vi "Register.vi"(5 "Color":T1={"Red"=0.0, "Green"=0.0, "Blue"=1.0, "Alpha"=1.0}, 6 "Point Size":sgl=10.0, 7 "Name":string, 8 "error in (no error)":errorcluster, 9 "Capacity":i32, 10 "Root Sence":refnum<vi>, 11 "Trace Drawer in":refnum<class "Trajectory Drawer.lvclass">) -> (0 "error out":errorcluster, 2 "Root Sence Out":refnum<vi>, 3 "Trace Drawer out":refnum<class "Trajectory Drawer.lvclass">)   [LabVIEW 2014, in "Trajectory Drawer.lvclass"]
uses:
  Trajectory Drawer.lvclass
  <vilib>/Utility/miscctls.llb/LVRGBAColorTypeDef.ctl
  Trajectory Drawer.lvclass/Trajectory Drawer.ctl
  <vilib>/picture/3D Picture Control/Object/Create Object (drawable with reference).vi
  <vilib>/picture/3D Picture Control/NI_3D Picture Control.lvlib
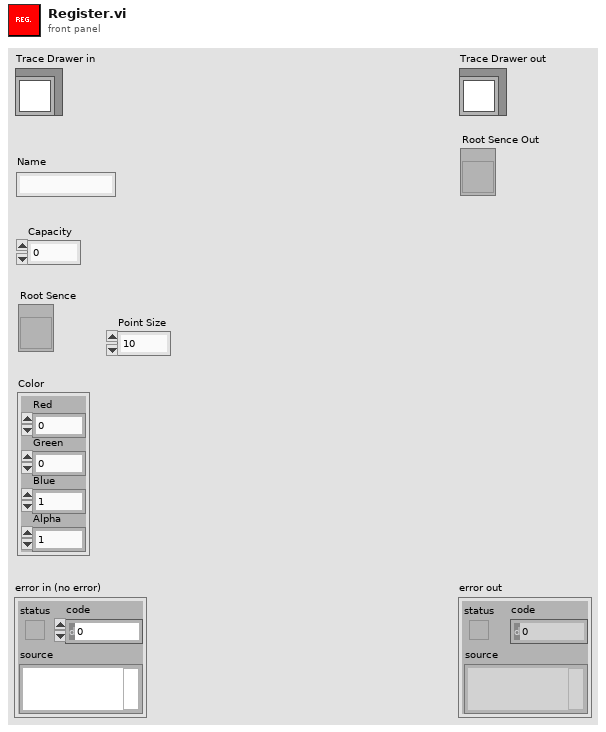
[diagram p1: front panel]
types:
  T1 = typedef "LVRGBAColorTypeDef.ctl" = cluster{"Red":sgl, "Green":sgl, "Blue":sgl, "Alpha":sgl}
  T2 = enum16{"Points", "Lines", "Line Strip", "Line Loop", "Triangles", "Triangle Strip", "Triangle Fan", "Quads", "Quad Strip", "Polygon"}
  T3 = enum16{"Overall", "Per Primitive", "Per Vertex", "Binding Off"}
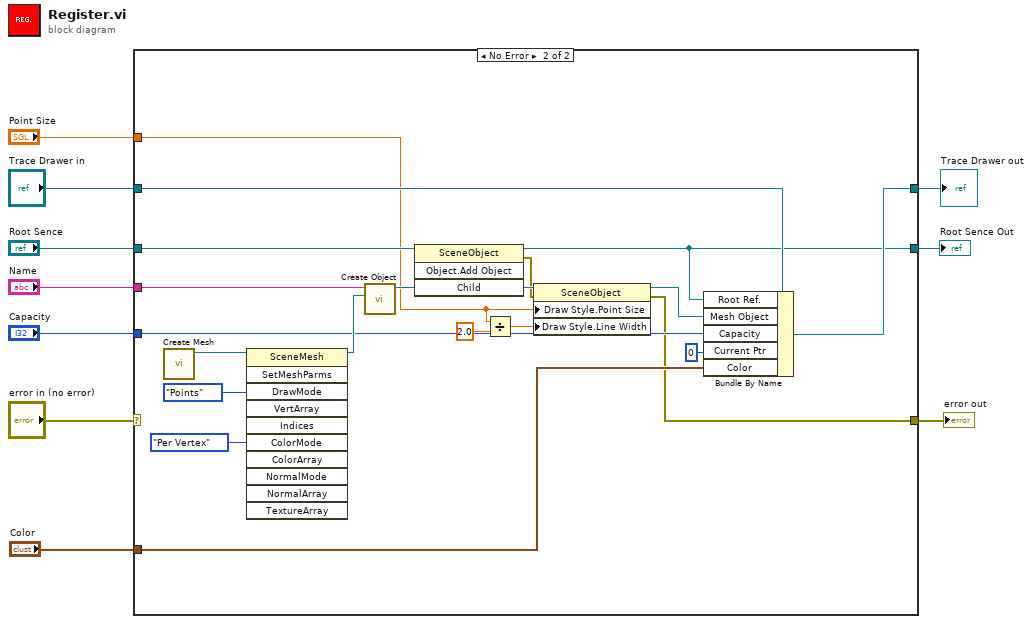
[diagram p0: block diagram]
diagram:
  n1 = case shown="No Error" "error in (no error)" {
    selector: "error in (no error)" -> [w12 _]
    tunnel: [w12 w17] -> w9
    tunnel: [w13 w31] -> w7
    tunnel: "Trace Drawer in" -> [w13 w27]
    tunnel: "Name" -> [_ w28]
    tunnel: "Capacity" -> [_ w26]
    tunnel: "Root Sence" -> [w11 w22]
    tunnel: "Color" -> [_ w24]
    tunnel: [w11 w21] -> w2
    tunnel: "Point Size" -> [_ w15]
    frame Error {
    }
    frame No Error {
      n2 = call <vilib>:"Create Mesh.vi"() -> ("New Mesh Refnum"=w33:refnum<vi>)  [unwired: 10 in, 1 out]
      n3 = invoke class="SceneMesh" method="SetMeshParms"(reference=w33, "DrawMode"=T2."Points" ("Draw Mode"), "ColorMode"=T3."Per Vertex" ("Color Binding Mode")) -> (reference out=w32:refnum<vi>)  [unwired: 8 in, 10 out]
      n4 = call-poly <vilib>:"Create Object.vi"("Geometry or text"=w32, "Name"=w28) -> ("Scene:New Object"=w23:refnum<vi>)  [unwired: 7 in, 2 out]
      n5 = invoke class="SceneObject" method="Object.Add Object"(reference=w22, "Child"=w23) -> (reference out=w21:refnum<vi>, error out=w18:errorcluster, "Child"=w20:refnum<vi>)  [unwired: 2 in, 1 out]
      n6 = Divide(x=w15, y=sgl 2.0) -> (x/y=w16:sgl)
      n7 = property class="SceneObject"(reference=w20, error in=w18, "Draw Style.Point Size"=w15, "Draw Style.Line Width"=w16) -> (reference out=w19:refnum<vi>, error out=w17:errorcluster)
      n8 = Bundle By Name(cluster=w27, "Root Ref."=w21, "Mesh Object"=w19, "Capacity"=w26, "Current Ptr"=0, "Color"=w24) -> (w31:refnum<class "Trajectory Drawer.lvclass">)
    }
  }
  "error out" <- w9
  "Trace Drawer out" <- w7
  "Root Sence Out" <- w2
